vi "RS_SMBV100A_DMS_TO_DEC.vi"(8 "error in":errorcluster {"code" format="%.0x"}, 11 "DMS":string) -> (0 "error out":errorcluster {"code" format="%.0x"}, 1 "hig":dbl, 2 "lon":dbl, 3 "lat":dbl)   [LabVIEW 2018]
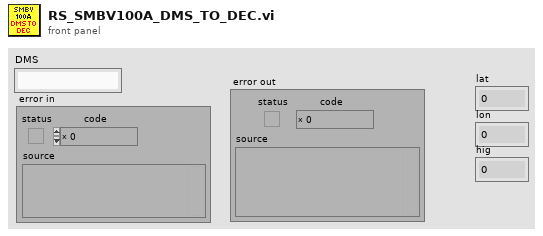
[diagram p1: front panel]
types:
  T1 = typedef "MLLC_Error.ctl" = errorcluster
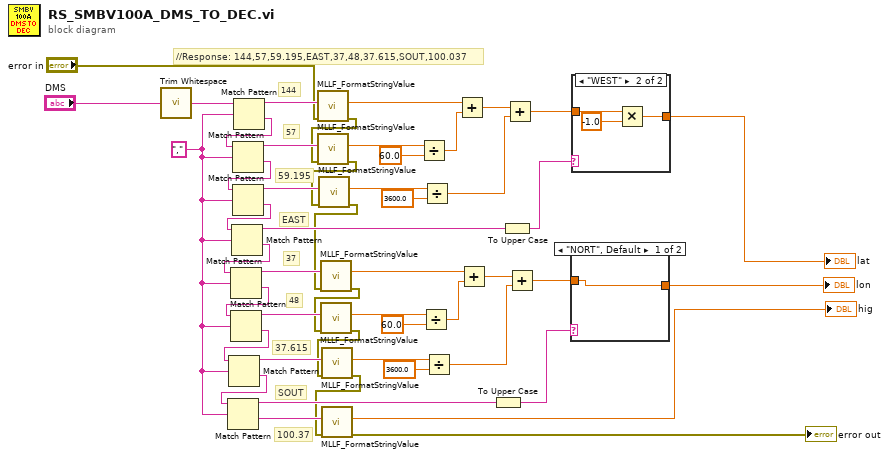
[diagram p0: block diagram]
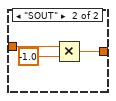
[diagram p2: hidden frame]
diagram:
  w39 = "," ("regular expression")
  # "100.37"
  # "SOUT"
  # "37.615"
  # "48"
  # "37"
  # "EAST"
  # "59.195"
  # "57"
  # "144"
  # "//Response: 144,57,59.195,EAST,37,48,37.615,SOUT,100.037"
  n1 = call <vilib>:"Trim Whitespace.vi"("string"="DMS") -> ("trimmed string"=w50:string)  [unwired: 1 in]
  n2 = Match Pattern(string=w50, regular expression=w39) -> (before substring=w48:string, after substring=w49:string)  [unwired: 1 in, 2 out]
  n3 = Match Pattern(string=w49, regular expression=w39) -> (before substring=w47:string, after substring=w45:string)  [unwired: 1 in, 2 out]
  n4 = Match Pattern(string=w45, regular expression=w39) -> (before substring=w46:string, after substring=w42:string)  [unwired: 1 in, 2 out]
  n5 = Match Pattern(string=w42, regular expression=w39) -> (before substring=w19:string, after substring=w44:string)  [unwired: 1 in, 2 out]
  n6 = Match Pattern(string=w44, regular expression=w39) -> (before substring=w38:string, after substring=w43:string)  [unwired: 1 in, 2 out]
  n7 = Match Pattern(string=w43, regular expression=w39) -> (before substring=w37:string, after substring=w40:string)  [unwired: 1 in, 2 out]
  n8 = Match Pattern(string=w40, regular expression=w39) -> (before substring=w36:string, after substring=w41:string)  [unwired: 1 in, 2 out]
  n9 = Match Pattern(string=w41, regular expression=w39) -> (before substring=w15:string, after substring=w13:string)  [unwired: 1 in, 2 out]
  n10 = call "MLLF_FormatStringValue.vi"("error in"="error in", "String Value"=w48) -> ("error out"=w12:T1, "number"=w35:dbl)  [unwired: 7 in, 1 out]
  n11 = call "MLLF_FormatStringValue.vi"("error in"=w12, "String Value"=w47) -> ("error out"=w11:T1, "number"=w34:dbl)  [unwired: 7 in, 1 out]
  n12 = call "MLLF_FormatStringValue.vi"("error in"=w11, "String Value"=w46) -> ("error out"=w10:T1, "number"=w30:dbl)  [unwired: 7 in, 1 out]
  n13 = call "MLLF_FormatStringValue.vi"("error in"=w10, "String Value"=w38) -> ("error out"=w9:T1, "number"=w22:dbl)  [unwired: 7 in, 1 out]
  n14 = call "MLLF_FormatStringValue.vi"("error in"=w9, "String Value"=w37) -> ("error out"=w8:T1, "number"=w21:dbl)  [unwired: 7 in, 1 out]
  n15 = call "MLLF_FormatStringValue.vi"("error in"=w8, "String Value"=w36) -> ("error out"=w7:T1, "number"=w20:dbl)  [unwired: 7 in, 1 out]
  n16 = call "MLLF_FormatStringValue.vi"("error in"=w7, "String Value"=w13) -> ("error out"=→"error out":T1, "number"=→"hig":dbl)  [unwired: 7 in, 1 out]
  n17 = Divide(x=w34, y=60.0) -> (x/y=w32:dbl)
  n18 = Divide(x=w21, y=60.0) -> (x/y=w26:dbl)
  n19 = Divide(x=w30, y=3600.0) -> (x/y=w29:dbl)
  n20 = Divide(x=w20, y=3600.0) -> (x/y=w24:dbl)
  n21 = Add(x=w35, y=w32) -> (x+y=w28:dbl)
  n22 = Add(x=w22, y=w26) -> (x+y=w23:dbl)
  n23 = To Upper Case(1:w15) -> (0:w14:string)
  n24 = To Upper Case(1:w19) -> (0:w18:string)
  n25 = Add(x=w28, y=w29) -> (x+y=w17:dbl)
  n26 = Add(x=w23, y=w24) -> (x+y=w16:dbl)
  n27 = case shown="\"NORT\", Default" w14 {
    tunnel: w16 -> [w51 w54]
    tunnel: [w51 w52] -> w2
    frame "NORT", Default {
    }
    frame "SOUT" {
      n28 = Multiply(x=w54, y=-1.0) -> (x*y=w52:dbl)
    }
  }
  "lon" <- w2
  n29 = case shown="\"WEST\"" w18 {
    tunnel: w17 -> [w55 w58]
    tunnel: [w55 w56] -> w3
    frame "EAST", Default {
    }
    frame "WEST" {
      n30 = Multiply(x=w58, y=-1.0) -> (x*y=w56:dbl)
    }
  }
  "lat" <- w3
